vi "UnBindControlFromMatlabValue.vi"(10 "Controls[]":refnum<vi>[](array[refnum]), 11 "Control":refnum<vi>) -> ()   [LabVIEW 2017]
panel:
  in  "ExpID":string
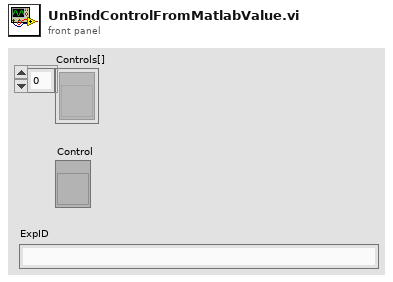
[diagram p1: front panel]
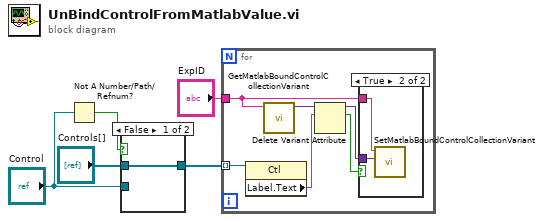
[diagram p0: block diagram]
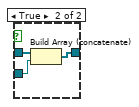
[diagram p3: hidden frame]
diagram:
  n1 = Not A Number/Path/Refnum?(number/path/refnum="Control") -> (NaN/Path/Refnum?=w5:bool)
  n2 = case shown="False" w5 {
    tunnel: "Controls[]" -> [w6 w9]
    tunnel: "Control" -> [_ w8]
    tunnel: [w6 w7] -> w2
    frame False {
    }
    frame True {
      n3 = Build Array (concatenate)(w9, w8) -> (w7:refnum<vi>[])
    }
  }
  n4 = for {
    tunnel: w2 -> [w12] mode=indexing
    tunnel: "ExpID" -> [w13]
    n5 = property class="Ctl"(reference=w12) -> ("Label.Text"=w11:string)  [unwired: 1 in, 2 out]
    n6 = call "GetMatlabBoundControlCollectionVariant.vi"("ExpID"=w13) -> ("BoundControlCollectionVariant"=w15:variant)  [unwired: 10 in]
    n7 = Delete Variant Attribute(6:w11, 7:w15) -> (2:w10:bool, 3:w14:variant)  [unwired: 1 in, 1 out]
    n8 = case shown="True" w10 {
      tunnel: w14 -> [_ w17]
      tunnel: w13 -> [_ w16]
      frame False {
      }
      frame True {
        n9 = call "SetMatlabBoundControlCollectionVariant.vi"("BoundControlCollectionVariant in"=w17, "ExpID"=w16) -> ()  [unwired: 9 in, 1 out]
      }
    }
  }
